vi "testClassInc.vi"(8 "error in (no error)":errorcluster caption="Fehler (Eingang, kein Fehler)", 11 "test Eingang":refnum<class "test.lvclass"> caption="DNL_LabVIEW Object in") -> (0 "error out":errorcluster caption="Fehler (Ausgang)", 3 "test Ausgang":refnum<class "test.lvclass"> caption="DNL_LabVIEW Object out")   [LabVIEW 2013, in "test.lvclass"]
uses:
  test.lvclass
  test.lvclass/test.ctl
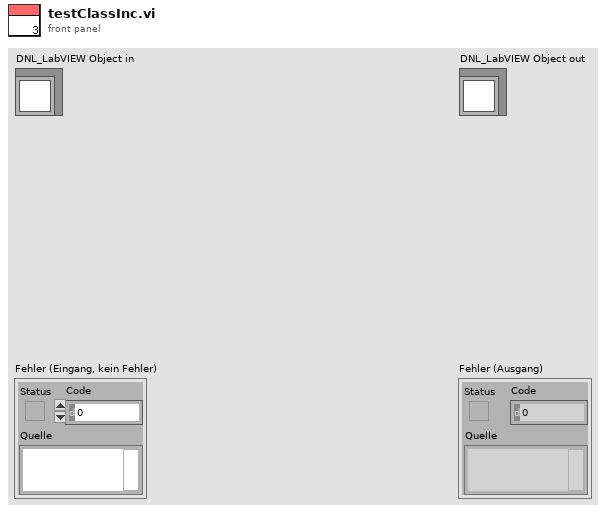
[diagram p1: front panel]
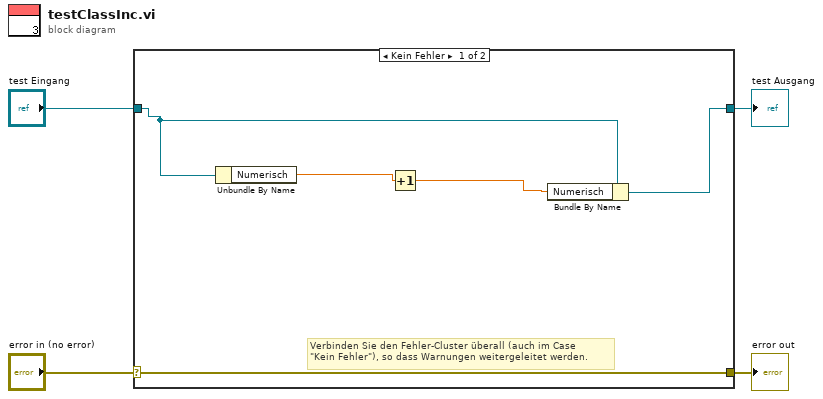
[diagram p0: block diagram]
diagram:
  n1 = case shown="Kein Fehler" "error in (no error)" {
    selector: "error in (no error)" -> [w9 w11]
    tunnel: [w9 w11] -> w3
    tunnel: [w8 w10] -> w1
    tunnel: "test Eingang" -> [w7 w10]
    frame No Error {
      # "Verbinden Sie den Fehler-Cluster überall (auch im Case\n\"Kein Fehler\"), so dass Warnungen weitergeleitet werden."
      n2 = Unbundle By Name(w7) -> ("Numerisch"=w6:dbl)
      n3 = Increment(x=w6) -> (x+1=w5:dbl)
      n4 = Bundle By Name(cluster=w7, "Numerisch"=w5) -> (w8:refnum<class "test.lvclass">)
    }
    frame Error {
    }
  }
  "error out" <- w3
  "test Ausgang" <- w1
